vi "SET_Show.vi"(8 "error in":errorcluster, 9 "Show Terminals?":bool, 11 "Settings.lvclass in":refnum<class "Settings.lvclass">) -> (0 "error out":errorcluster, 3 "Settings.lvclass out":refnum<class "Settings.lvclass">)   [LabVIEW 2020, in "Settings.lvclass"]
uses:
  Settings.lvclass
  Settings.lvclass/Settings.ctl
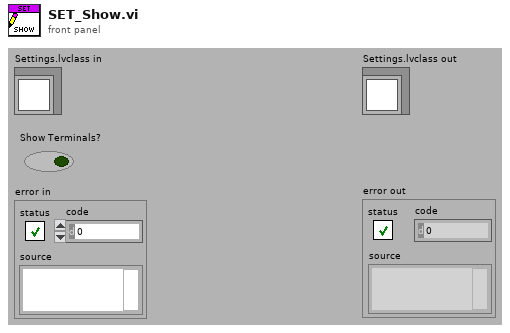
[diagram p1: front panel]
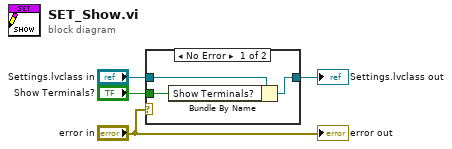
[diagram p0: block diagram]
diagram:
  n1 = case shown="No Error" "error in" {
    tunnel: [w6 w8] -> w2
    tunnel: "Settings.lvclass in" -> [w7 w8]
    tunnel: "Show Terminals?" -> [w5 _]
    frame No Error {
      n2 = Bundle By Name(cluster=w7, "Show Terminals?"=w5) -> (w6:refnum<class "Settings.lvclass">)
    }
    frame Error {
    }
  }
  "Settings.lvclass out" <- w2
  "error out" <- "error in"
